vi "I2C.vi"() -> ()   [LabVIEW 2017]
uses:
  <vilib>/myRIO/Instrument Drivers/Onboard IO/I2C/typedefs/I2C User Configuration.ctl
  <vilib>/myRIO/Instrument Drivers/Onboard IO/I2C/typedefs/I2C Transfer Rate.ctl
  <vilib>/myRIO/Common/Instrument Driver Framework/myRIO v1.0/Resource Manager/vis/myRIO v1.0 Unreserve Channel List.vi
  <vilib>/myRIO/Common/Instrument Driver Framework/myRIO v1.0/Resource Manager/vis/myRIO v1.0 Create Configuration List.vi
  <vilib>/myRIO/Common/Instrument Driver Framework/myRIO v1.0/Resource Manager/vis/myRIO v1.0 Unreserve Channel.vi
  <vilib>/myRIO/Common/Instrument Driver Framework/myRIO v1.0/Resource Manager/vis/myRIO v1.0 Build Mutex Name.vi
  <vilib>/Utility/error.llb/Error Cluster From Error Code.vi
  <vilib>/myRIO/Common/Instrument Driver Framework/myRIO v1.0/Resource Manager/vis/myRIO v1.0 Configure IO.vi
  <vilib>/myRIO/Common/Instrument Driver Framework/Utilities/vis/Configuration Manager.vi
  <vilib>/myRIO/Common/Instrument Driver Framework/Utilities/vis/IO Manager.vi
  <vilib>/myRIO/Common/Instrument Driver Framework/myRIO v1.0/myRIO v1.0 Close.vi
  <vilib>/myRIO/Instrument Drivers/Onboard IO/I2C/I2C.lvlib
panel:
  in  "Stop Button":bool
  out "Voltage(mv)":dbl
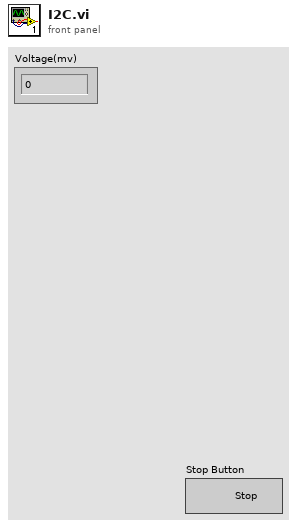
[diagram p1: front panel]
types:
  T1 = typedef "I2C.lvlib/I2C User Configuration.ctl" = cluster{"I2C Transfer Rate":T2}
  T2 = typedef "I2C.lvlib/I2C Transfer Rate.ctl" = enum16{"Standard mode (100 kbps)", "Fast mode (400 kbps)"}
  T3 = typedef "I2C.lvlib/I2C Reference.ctl" = cluster{"myRIO Reference":T4, "I2C Channels Enum":T8, "I2C Configuration":T9}
  T4 = typedef "myRIO Generic Hardware Reference.ctl" = cluster{"myRIO Model":T5, "myRIO Hardware Reference":T6}
  T5 = typedef "Hardware Version Enum.ctl" = enum16{"Unknown", "myRIO-1900", "myRIO-1950", "roboRIO", "NI ELVIS RIO CM"}
  T6 = typedef "myRIO v1.0 Reference.ctl" = cluster{"Generic FPGA Reference":T7, "Allow multiple opens":bool}
  T7 = typedef "Generic FPGA Reference.ctl" = refnum<k20>
  T8 = typedef "I2C Channels Enum.ctl" = enum16{"Not Connected", "A/I2C", "B/I2C", "I2C/I2C"}
  T9 = typedef "I2C.lvlib/I2C Configuration.ctl" = cluster{"I2C Transfer Rate":T2}
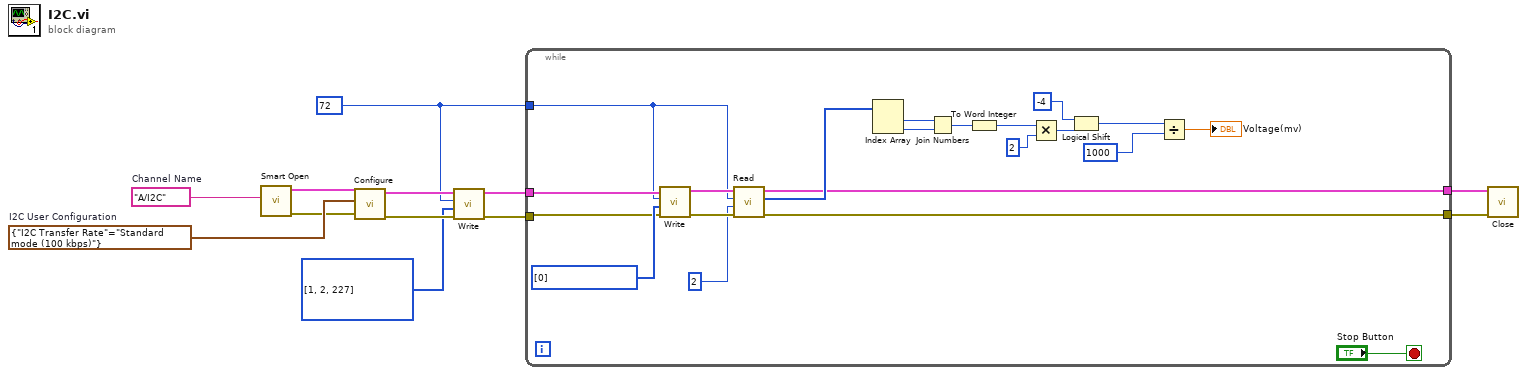
[diagram p0: block diagram]
diagram:
  w11 = tag "A/I2C"  # Channel Name
  w12 = T1 {"I2C Transfer Rate"=enum."Standard mode (100 kbps)"}  # I2C User Configuration
  w3 = 72 ("I2C Slave Address (0)")
  n1 = call <vilib>:"Smart Open.vi"("Channel Name"=w11) -> ("error out"=w9:errorcluster, "I2C Ref Out"=w10:T3)  [unwired: 9 in]
  n2 = call <vilib>:"Configure.vi"("error in (no error)"=w9, "I2C User Configuration"=w12, "I2C Ref In"=w10) -> ("error out"=w7:errorcluster, "I2C Ref Out"=w8:T3)  [unwired: 7 in]
  n3 = call <vilib>:"Write.vi"("error in (no error)"=w7, "Bytes to Write"=u8[] [1, 2, 227] ("Data"), "Slave Address (7-bit)"=w3, "I2C Ref In"=w8) -> ("error out"=w4:errorcluster, "I2C Ref Out"=w5:T3)  [unwired: 6 in]
  n4 = while {
    tunnel: w5 -> [w19]
    tunnel: w4 -> [w18]
    tunnel: w3 -> [w14]
    tunnel: [w16] -> w2
    tunnel: [w15] -> w1
    stop <- "Stop Button" stop-if-true
    n5 = call <vilib>:"Write.vi"("error in (no error)"=w18, "Bytes to Write"=u8[] [0] ("Data"), "Slave Address (7-bit)"=w14, "I2C Ref In"=w19) -> ("error out"=w21:errorcluster, "I2C Ref Out"=w22:T3)  [unwired: 6 in]
    n6 = call <vilib>:"Read.vi"("error in (no error)"=w21, "Byte Count"=u8 2 ("Bytes To Read"), "Slave Address (7-bit)"=w14, "I2C Ref In"=w22) -> ("error out"=w15:errorcluster, "Bytes Read"=w17:u8[], "I2C Ref Out"=w16:T3)  [unwired: 4 in]
    n7 = Index Array(array=w17) -> (element #1=w33:u8, element #2=w32:u8)  [unwired: 2 in]
    n8 = Join Numbers(hi=w33, lo=w32) -> ((hi.lo)=w31:u16)
    n9 = To Word Integer(number=w31) -> (16bit integer=w30:i16)
    n10 = Multiply(x=w30, y=i16 2) -> (x*y=w28:i16)
    n11 = Logical Shift(y=i16 -4, x=w28) -> (x << y=w25:i16)
    n12 = Divide(x=w25, y=i16 1000) -> (x/y=→"Voltage(mv)":dbl)
  }
  n13 = call <vilib>:"Close.vi"("error in (no error)"=w1, "I2C Ref In"=w2) -> ()  [unwired: 9 in, 1 out]
